vi "Close FITS Reference.vi"(8 "error in (no error)":errorcluster, 11 "Save Image in":refnum<class "Save Image.lvclass">) -> (0 "error out":errorcluster, 3 "Save Image out":refnum<class "Save Image.lvclass">)   [LabVIEW 2018, in "Save Image.lvclass"]
uses:
  Save Image.lvclass
  Save Image.lvclass/Save Image.ctl
  <userlib>/gfitsio/gfitsio.lvlib
  Simulated_Header/Simulated_Header.lvclass
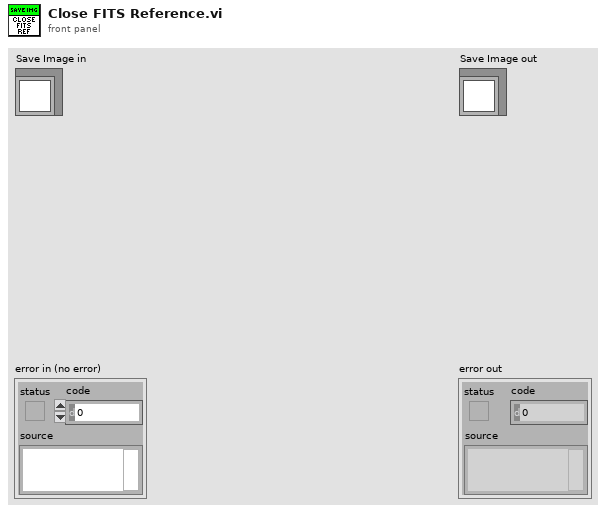
[diagram p1: front panel]
types:
  T1 = typedef "gfitsio.lvlib/gfitsio-refnum.ctl" = refnum<k1>
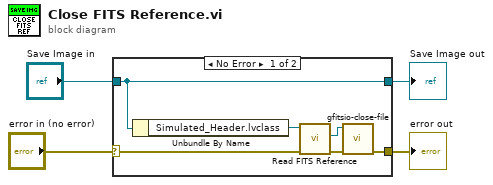
[diagram p0: block diagram]
diagram:
  n1 = case shown="No Error" "error in (no error)" {
    selector: "error in (no error)" -> [w5 w12]
    tunnel: [w10 w12] -> w3
    tunnel: [w7 w11] -> w1
    tunnel: "Save Image in" -> [w7 w11]
    frame No Error {
      n2 = Unbundle By Name(w7) -> ("Simulated_Header.lvclass"=w6:refnum<class "Simulated_Header.lvclass">)
      n3 = call "Read FITS Reference.vi"("error in (no error)"=w5, "Simulated_Header in"=w6) -> ("error out"=w9:errorcluster, "gfits refnum"=w8:T1)  [unwired: 7 in, 1 out]
      n4 = call <userlib>:"gfitsio-close-file.vi"("error in (no error)"=w9, "gfits refnum"=w8) -> ("error out"=w10:errorcluster)  [unwired: 8 in, 1 out]
    }
    frame Error {
    }
  }
  "error out" <- w3
  "Save Image out" <- w1
